vi "Read Sample Transfer State.vi"(8 "error in (no error)":errorcluster, 9 "State Timeout (Inf)":dbl=inf, 10 "Reinit Timer (F)":bool caption="Reset", 11 "cRIO-CO2 in":refnum<class "cRIO-CO2.lvclass">) -> (0 "error out":errorcluster, 1 "Sample Transfer State":string, 2 "Sample Transfer State":T1, 3 "cRIO-CO2 out":refnum<class "cRIO-CO2.lvclass">, 4 "Timeout?":bool, 6 "Elapsed Time (s)":dbl)   [LabVIEW 2015, in "cRIO-Carbondioxide.lvlib" / "cRIO-CO2.lvlib" / "cRIO-CO2.lvclass"]
uses:
  cRIO-CO2.lvclass
  Controls/Sample Transfer State Enumerator.ctl
  cRIO-CO2.lvclass/cRIO-CO2.ctl
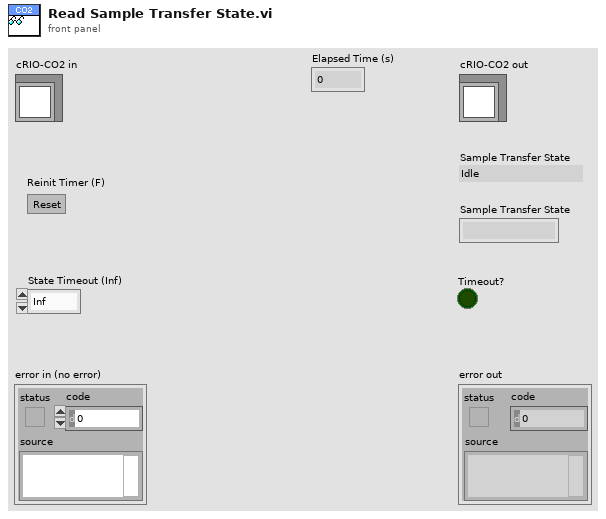
[diagram p1: front panel]
types:
  T1 = typedef "Sample Transfer State Enumerator.ctl" = enum16{"Idle", "Initialize", "Check Containers", "Check Temperatures", "Start Turbo", "Warm Up Containers", "Prepare for purging", "Purge Capillary", "Purge", "Open Containers", "Introduce Sample", "Measure Base Pressure", "Home Syringe", "Start Freezer", "Freeze Target", "Crystalize", "Initiate Stash", "Stash", "Polish", "Stop Freezers", "Push Sample", "Complete", "Abort", "Error", "Undefined"}
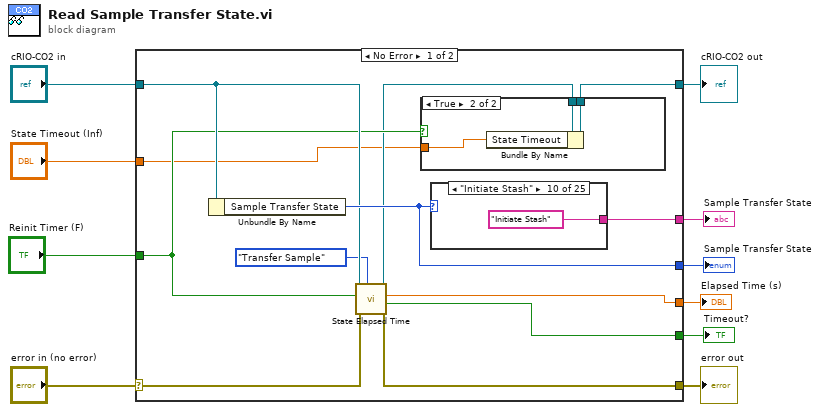
[diagram p0: block diagram]
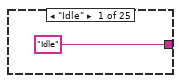
[diagram p3: hidden frame]
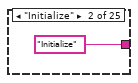
[diagram p4: hidden frame]
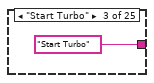
[diagram p5: hidden frame]
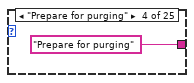
[diagram p6: hidden frame]
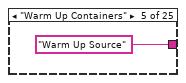
[diagram p7: hidden frame]
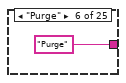
[diagram p8: hidden frame]
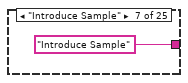
[diagram p9: hidden frame]
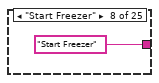
[diagram p10: hidden frame]
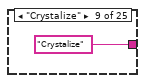
[diagram p11: hidden frame]
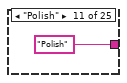
[diagram p12: hidden frame]
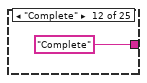
[diagram p13: hidden frame]
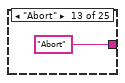
[diagram p14: hidden frame]
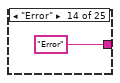
[diagram p15: hidden frame]
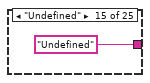
[diagram p16: hidden frame]
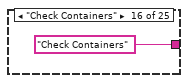
[diagram p17: hidden frame]
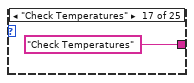
[diagram p18: hidden frame]
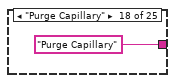
[diagram p19: hidden frame]
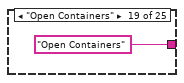
[diagram p20: hidden frame]
diagram:
  n1 = case shown="No Error" "error in (no error)" {
    selector: "error in (no error)" -> [w18 w53]
    tunnel: [w17 w53] -> w9
    tunnel: [w14 w54] -> w7
    tunnel: "cRIO-CO2 in" -> [w19 w54]
    tunnel: [w21 _] -> w6
    tunnel: [w22 "Undefined"] -> w5
    tunnel: [w20 _] -> w4
    tunnel: "Reinit Timer (F)" -> [w16 _]
    tunnel: "State Timeout (Inf)" -> [w13 _]
    tunnel: [w11 _] -> w1
    frame No Error {
      n2 = Unbundle By Name(w19) -> ("Sample Transfer State"=w21:T1)
      n3 = call "State Elapsed Time.vi"("State Machine"=enum16{"Transfer Sample", "Push Sample"}."Transfer Sample", "error in (no error)"=w18, "Reset (F)"=w16, "cRIO-CO2 in"=w19) -> ("error out"=w17:errorcluster, "State Timeout?"=w20:bool, "Elapsed Time (s)"=w11:dbl, "cRIO-CO2 out"=w15:refnum<class "cRIO-CO2.lvclass">)  [unwired: 4 in]
      n4 = case shown="True" w16 {
        tunnel: w15 -> [w23 w26]
        tunnel: [w23 w25] -> w14
        tunnel: w13 -> [_ w24]
        frame False {
        }
        frame True {
          n5 = Bundle By Name(cluster=w26, "State Timeout"=w24) -> (w25:refnum<class "cRIO-CO2.lvclass">)
        }
      }
      n6 = case shown="\"Initiate Stash\"" w21 {
        tunnel: ["Idle" "Initialize" "Start Turbo" "Prepare for purging" "Warm Up Source" "Purge" "Introduce Sample" "Start Freezer" "Crystalize" "Initiate Stash" "Polish" "Complete" "Abort" "Error" "Undefined" "Check Containers" "Check Temperatures" "Purge Capillary" "Open Containers" "Measure Base Pressure" "Home Syringe" "Stash" "Stop Freezerz" "Push Sample" "Freeze Target"] -> w22
        frame "Idle" {
        }
        frame "Initialize" {
        }
        frame "Start Turbo" {
        }
        frame "Prepare for purging" {
        }
        frame "Warm Up Containers" {
        }
        frame "Purge" {
        }
        frame "Introduce Sample" {
        }
        frame "Start Freezer" {
        }
        frame "Crystalize" {
        }
        frame "Initiate Stash" {
        }
        frame "Polish" {
        }
        frame "Complete" {
        }
        frame "Abort" {
        }
        frame "Error" {
        }
        frame "Undefined" {
        }
        frame "Check Containers" {
        }
        frame "Check Temperatures" {
        }
        frame "Purge Capillary" {
        }
        frame "Open Containers" {
        }
        frame "Measure Base Pressure" {
        }
        frame "Home Syringe" {
        }
        frame "Stash" {
        }
        frame "Stop Freezers" {
        }
        frame "Push Sample" {
        }
        frame "Freeze Target" {
        }
      }
    }
    frame Error {
    }
  }
  "error out" <- w9
  "cRIO-CO2 out" <- w7
  "Sample Transfer State" <- w6
  "Sample Transfer State" <- w5
  "Timeout?" <- w4
  "Elapsed Time (s)" <- w1
